vi "Get Status.vi"(8 "error in (no error)":errorcluster, 10 "Light Selection":T1, 11 "LightsPanel in":refnum<class "LightsPanel.lvclass">) -> (0 "error out":errorcluster, 1 "Temperature":dbl, 2 "Brightness":i32, 3 "LightsPanel out":refnum<class "LightsPanel.lvclass">, 5 "On":bool)   [LabVIEW 2022 SP3, in "TouchControl.lvlib" / "LightsPanel.lvclass"]
uses:
  LightsPanel.lvclass
  Light Selection.ctl
  TouchControl.lvlib
  <vilib>/httpClient/LabVIEWHTTPClient.lvlib
  <vilib>/IlluminatedG/lv-web-crypto/lv-json/JSON/JSON.lvlib
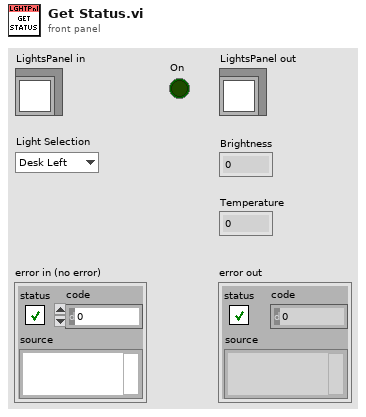
[diagram p1: front panel]
types:
  T1 = typedef "TouchControl.lvlib/Light Selection.ctl" = enum16{"Desk Left", "Desk Right", "Printer"}
  T2 = typedef "TouchControl.lvlib/Light Config.ctl" = cluster{"Desk Left":string, "Desk Right":string, "Printer":string}
  T3 = typedef "JSON.lvlib/JSON Item Type.ctl" = enum16{"unknown", "null", "Array", "Object", "String", "Number", "Boolean"}
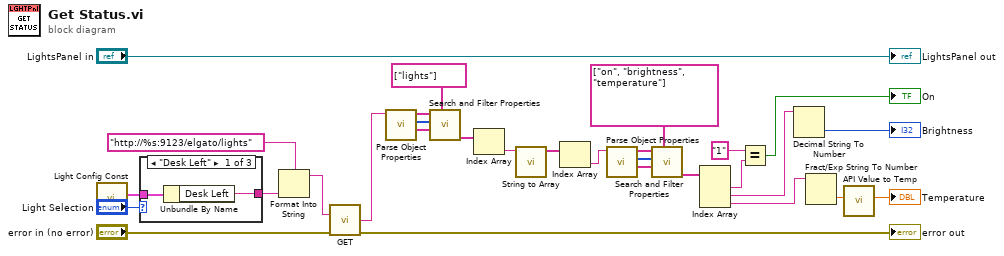
[diagram p0: block diagram]
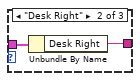
[diagram p2: hidden frame]
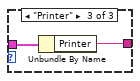
[diagram p3: hidden frame]
diagram:
  n1 = call "Light Config Const.vi"() -> ("Light Config"=w29:T2)  [unwired: 11 in]
  n2 = case shown="\"Desk Left\"" "Light Selection" {
    tunnel: w29 -> [w32 w34 w36]
    tunnel: [w31 w33 w35] -> w24
    frame "Desk Left" {
      n3 = Unbundle By Name(w32) -> ("Desk Left"=w31:string)
    }
    frame "Desk Right" {
      n4 = Unbundle By Name(w34) -> ("Desk Right"=w33:string)
    }
    frame "Printer" {
      n5 = Unbundle By Name(w36) -> ("Printer"=w35:string)
    }
  }
  n6 = Format Into String(format string="http://%s:9123/elgato/lights", w24) -> (resulting string=w22:string)  [unwired: 2 in, 1 out]
  n7 = call <vilib>:"GET.vi"("url"=w22, "error in (no error)"="error in (no error)") -> ("body"=w25:string, "error out"=→"error out":errorcluster)  [unwired: 10 in, 2 out]
  n8 = call <vilib>:"Parse Object Properties.vi"("JSON String"=w25) -> ("Values"=w19:string[], "Item Types"=w20:T3[], "Keys"=w21:string[])  [unwired: 7 in, 1 out]
  n9 = call <vilib>:"Search and Filter Properties.vi"("Search Keys"=string[] ["lights"], "Values In"=w19, "Types In"=w20, "Keys In"=w21) -> ("Filtered Values"=w17:string[])  [unwired: 2 in, 5 out]
  n10 = Index Array(array=w17) -> (element=w3:string)  [unwired: 1 in]
  n11 = call <vilib>:"String to Array.vi"("Array String In"=w3) -> ("JSON Strings"=w2:string[])  [unwired: 10 in]
  n12 = Index Array(array=w2) -> (element=w1:string)  [unwired: 1 in]
  n13 = call <vilib>:"Parse Object Properties.vi"("JSON String"=w1) -> ("Values"=w14:string[], "Item Types"=w15:T3[], "Keys"=w16:string[])  [unwired: 7 in, 1 out]
  n14 = call <vilib>:"Search and Filter Properties.vi"("Search Keys"=string[] ["on", "brightness", "temperature"], "Values In"=w14, "Types In"=w15, "Keys In"=w16) -> ("Filtered Values"=w12:string[])  [unwired: 2 in, 5 out]
  n15 = Index Array(array=w12) -> (element #1=w11:string, element #2=w8:string, element #3=w6:string)  [unwired: 3 in]
  n16 = Equal?(x="1", y=w11) -> (x = y?=→"On":bool)
  n17 = Decimal String To Number(string=w8) -> (number=→"Brightness":i32)  [unwired: 2 in, 1 out]
  n18 = Fract/Exp String To Number(string=w6) -> (number=w5:dbl)  [unwired: 3 in, 1 out]
  n19 = call "API Value to Temp.vi"("API Temp"=w5) -> ("Color Temp"=→"Temperature":dbl)  [unwired: 10 in]
  "LightsPanel out" <- "LightsPanel in"
